vi "Fir_reloadable.vi"(6 "reset":bool, 7 "Coeffs":fxp<+/-,18,18>[](array[numeric]), 8 "valid in":bool, 9 "Q in":fxp<+/-,25,19>, 10 "I in":fxp<+/-,25,19>, 11 "new coeffs":bool) -> (0 "valid out":bool, 1 "Q out":fxp<+/-,16,16>, 2 "I out":fxp<+/-,16,16>, 4 "ready for input":bool)   [LabVIEW 2013]
uses:
  <vilib>/rvi/XilinxIP/XIPIN_XNode/niFpgaXIPIN.xnode
  <vilib>/rvi/FXPMathLib/FxpInterpret/XNode/nifxpmath_Interpret.xnode
  <vilib>/fxp/LVFixedPointOverflowPolicyTypeDef.ctl
  <vilib>/fxp/LVFixedPointQuantizationPolicyTypeDef.ctl
  <vilib>/rvi/FXPMathLib/FxpConvert/subVIs/nifxpmath_Convert_SimConfig.ctl
  <vilib>/rvi/FXPMathLib/FxpConvert/simVIs/DllFxpConvertTemp_sub.vi
  <vilib>/rvi/FXPMathLib/FxpConvert/XNode/nifxpmath_Convert.xnode
  Xilinx compiled/FIR_reload/FIR_configurable_8932671C180D4D8FA00E62E84E1DBB19.dll
  <vilib>/rvi/IPIntegrationNode/IPINode_Xnode/niFpgaIPINode.xnode
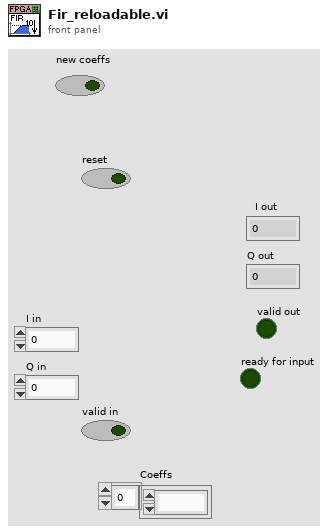
[diagram p1: front panel]
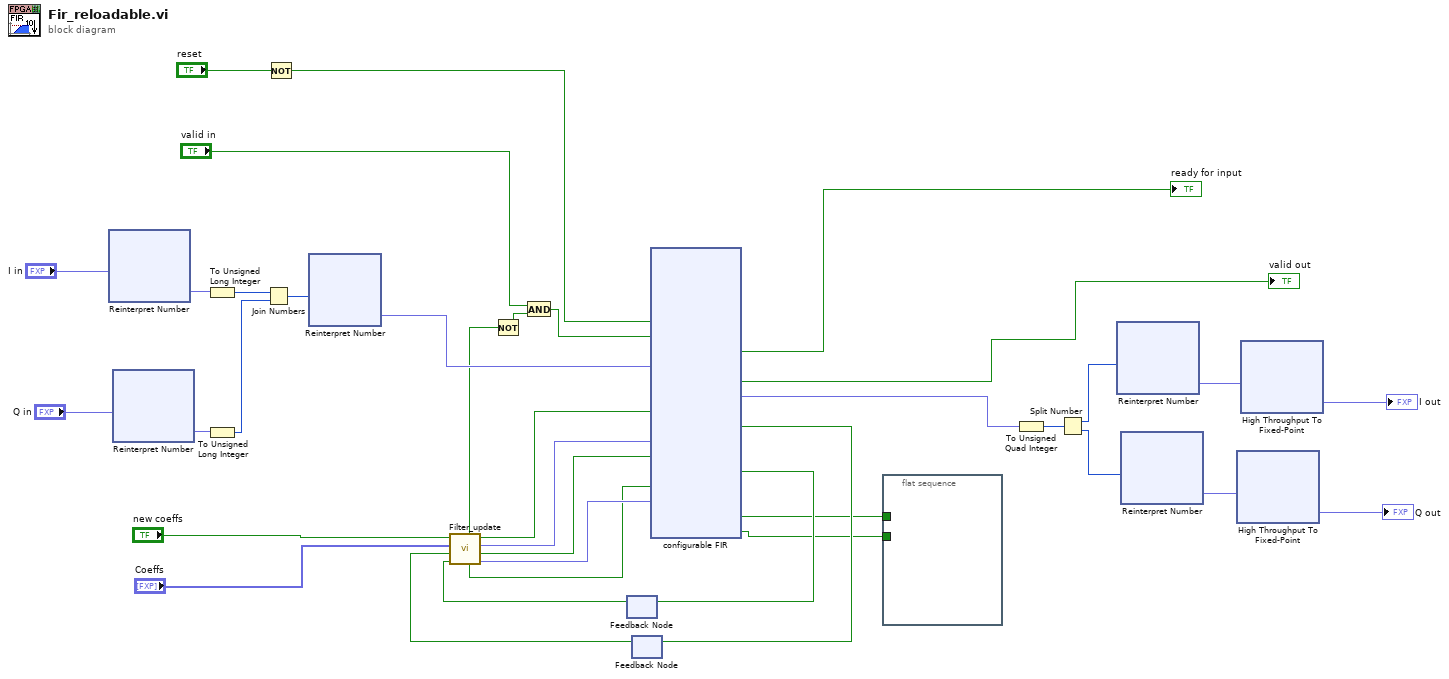
[diagram p0: block diagram]
diagram:
  n1 = xnode "Reinterpret Number"("x"="I in") -> ("y"=w34:fxp<+,25,25>)
  n2 = xnode "Reinterpret Number"("x"="Q in") -> ("y"=w36:fxp<+,25,25>)
  n3 = To Unsigned Long Integer(number=w34) -> (unsigned 32bit integer=w35:u32)
  n4 = To Unsigned Long Integer(number=w36) -> (unsigned 32bit integer=w37:u32)
  n5 = Join Numbers(hi=w35, lo=w37) -> ((hi.lo)=w31:u64)
  n6 = Not(x="reset") -> (.not. x?=w22:bool)
  n7 = xnode "Reinterpret Number"("x"=w31) -> ("y"=w18:fxp<+,64,64>)
  n8 = feedback #1() -> (w16:bool)  [unwired: 1 in]
  n9 = feedback #2() -> (w12:bool)  [unwired: 1 in]
  n10 = call "Filter_update.vi"("reload rdy for data"=w16, "config rdy for data"=w12, "Coeffs"="Coeffs", "new coeffs"="new coeffs") -> ("s_axis_reload_tdata"=w10:fxp<+,24,24>, "s_axis_reload_tvalid"=w11:bool, "s_axis_config_tdata"=w14:fxp<+,8,8>, "s_axis_config_tvalid"=w15:bool, "s_axis_reload_tlast"=w9:bool, "busy"=w4:bool)  [unwired: 2 in]
  n11 = Not(x=w4) -> (.not. x?=w3:bool)
  n12 = And(x="valid in", y=w3) -> (x .and. y?=w1:bool)
  n13 = xnode "configurable FIR"("aresetn"=w22, "s_axis_data_tvalid"=w1, "s_axis_data_tdata"=w18, "s_axis_config_tvalid"=w15, "s_axis_config_tdata"=w14, "s_axis_reload_tvalid"=w11, "s_axis_reload_tlast"=w9, "s_axis_reload_tdata"=w10) -> ("s_axis_data_tready"=→"ready for input":bool, "m_axis_data_tvalid"=→"valid out":bool, "m_axis_data_tdata"=w19:fxp<+,64,64>, "s_axis_config_tready"=w13:bool, "s_axis_reload_tready"=w17:bool, "event_s_reload_tlast_missing"=w6:bool, "event_s_reload_tlast_unexpected"=w5:bool)  [unwired: 1 in]
  n14 = feedback-in #1(w17) -> ()
  n15 = feedback-in #2(w13) -> ()
  n16 = flat-sequence {
    tunnel: w6 -> [_]
    tunnel: w5 -> [_]
    frame #0 {
    }
  }
  n17 = To Unsigned Quad Integer(1:w19) -> (0:w26:u64)
  n18 = Split Number(x=w26) -> (hi(x)=w25:u32, lo(x)=w24:u32)
  n19 = xnode "Reinterpret Number"("x"=w25) -> ("y"=w28:fxp<+/-,32,20>)
  n20 = xnode "Reinterpret Number"("x"=w24) -> ("y"=w27:fxp<+/-,32,20>)
  n21 = xnode "High Throughput To Fixed-Point"("x"=w27) -> ("y"=→"Q out":fxp<+/-,16,16>)
  n22 = xnode "High Throughput To Fixed-Point"("x"=w28) -> ("y"=→"I out":fxp<+/-,16,16>)
